vi "subXMLFindAndDeleteNodeFromName.vi"(9 "Property value":string, 10 "Property name":string, 11 "Refnum in":refnum<k20>) -> (0 "error out":errorcluster, 2 "Found?":bool, 3 "Refnum out":refnum<k20>)   [LabVIEW 2019]
uses:
  <resource>/objmgr/DOMUserDefRef.rc
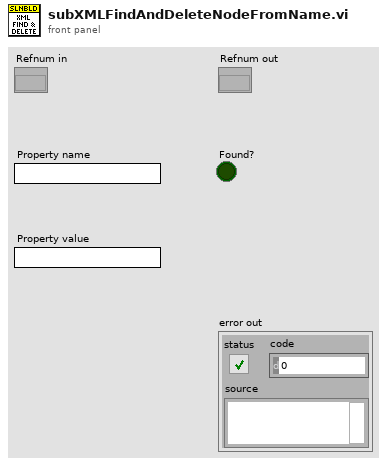
[diagram p1: front panel]
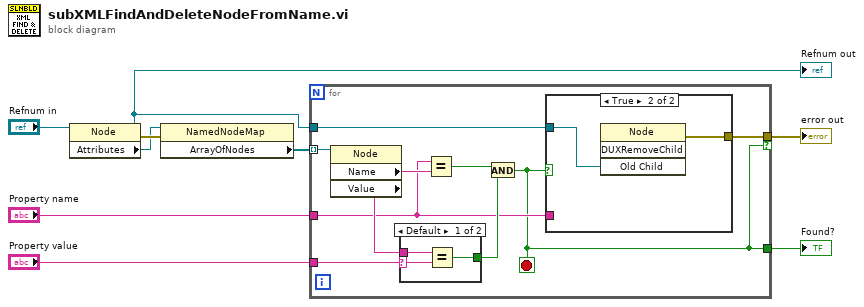
[diagram p0: block diagram]
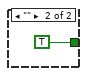
[diagram p3: hidden frame]
diagram:
  n1 = property class="Node"(reference="Refnum in") -> (reference out=w1:refnum<k20>, error out=w5:errorcluster, "Attributes"=w3:refnum<k20>)  [unwired: 1 in]
  "Refnum out" <- w1
  n2 = property class="NamedNodeMap"(reference=w3, error in=w5) -> ("ArrayOfNodes"=w4:refnum<k20>[])  [unwired: 2 out]
  n3 = for {
    tunnel: w4 -> [w19] mode=indexing
    tunnel: [w10] -> w9
    tunnel: "Property name" -> [w12]
    tunnel: "Property value" -> [w15]
    tunnel: w1 -> [w13]
    tunnel: [w11] -> w2 if=w10
    stop <- w10 stop-if-true
    n4 = property class="Node"(reference=w19) -> ("Name"=w14:string, "Value"=w16:string)  [unwired: 1 in, 2 out]
    n5 = case shown="Default" w15 {
      selector: w15 -> [w22 _]
      tunnel: [w24 TRUE] -> w17
      tunnel: w16 -> [w23 _]
      frame Default {
        n6 = Equal?(x=w23, y=w22) -> (x = y?=w24:bool)
      }
      frame "" {
      }
    }
    n7 = Equal?(x=w12, y=w14) -> (x = y?=w18:bool)
    n8 = And(x=w18, y=w17) -> (x .and. y?=w10:bool)
    n9 = case shown="True" w10 {
      tunnel: w13 -> [_ w20]
      tunnel: w12 -> [_ _]
      tunnel: [_ w21] -> w11
      frame False {
      }
      frame True {
        n10 = invoke class="Node" method="DUXRemoveChild"("Old Child"=w20) -> (error out=w21:errorcluster)  [unwired: 3 in, 3 out]
      }
    }
  }
  "Found?" <- w9
  "error out" <- w2
